vi "temp state machine(SUB).vi"() -> ()   [LabVIEW 2012]
panel:
  out "Enum":enum16{"High", "Medium", "low"}(ring)
  in  "Boolean":bool
  in  "stop":bool
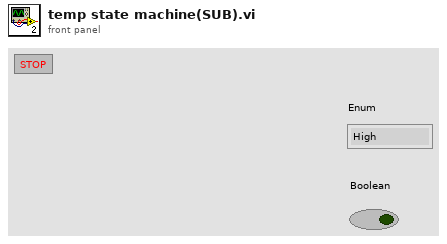
[diagram p1: front panel]
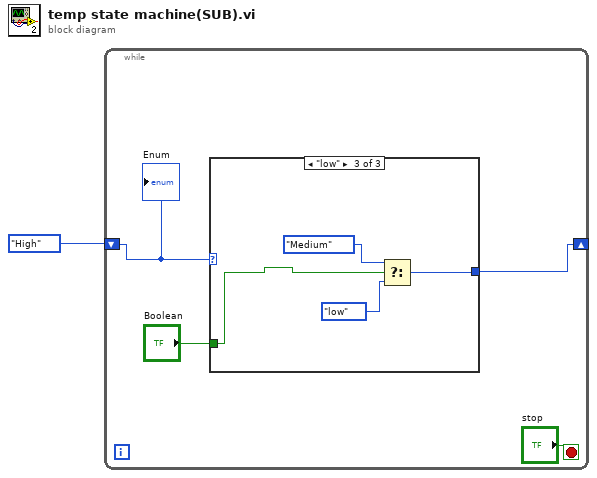
[diagram p0: block diagram]
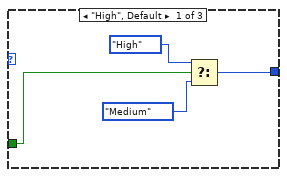
[diagram p2: hidden frame]
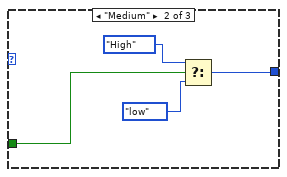
[diagram p3: hidden frame]
diagram:
  n1 = while {
    shift-right: [w3] -> _
    shift-left: enum16{"High", "Medium", "low"}."High" ("Enum") -> [w2]
    stop <- "stop" stop-if-true
    n2 = case shown="\"low\"" w2 {
      tunnel: "Boolean" -> [w6 w13 w14]
      tunnel: [w7 w10 w15] -> w3
      frame "High", Default {
        n3 = Select(t=enum16{"High", "Medium", "low"}."High" ("Enum"), s=w6, f=enum16{"High", "Medium", "low"}."Medium" ("Enum")) -> (s? t:f=w7:enum16{"High", "Medium", "low"})
      }
      frame "Medium" {
        n4 = Select(t=enum16{"High", "Medium", "low"}."High" ("Enum"), s=w13, f=enum16{"High", "Medium", "low"}."low" ("Enum")) -> (s? t:f=w10:enum16{"High", "Medium", "low"})
      }
      frame "low" {
        n5 = Select(t=enum16{"High", "Medium", "low"}."Medium" ("Enum"), s=w14, f=enum16{"High", "Medium", "low"}."low" ("Enum")) -> (s? t:f=w15:enum16{"High", "Medium", "low"})
      }
    }
    "Enum" <- w2
  }
